vi "Get Daemon Error.vi"(8 "error in (no error)":errorcluster, 11 "Modbus slave in":refnum<class "Modbus Slave.lvclass">) -> (0 "error out":errorcluster, 2 "daemon error":errorcluster, 3 "Modbus Slave out":refnum<class "Modbus Slave.lvclass">)   [LabVIEW 2013, in "Modbus Library - Advance.lvlib" / "Modbus Slave.lvclass"]
doc: "This VI is an accessor for the <B>daemon error</B> stored in the Modbus slave instance. This accessor can be used as a property node. This status indicates the error state of the Modbus daemon."
uses:
  Modbus Slave.lvclass
  Modbus Slave.lvclass/Modbus Slave.ctl
  Network Protocol/Network Slave/Network Slave.lvclass
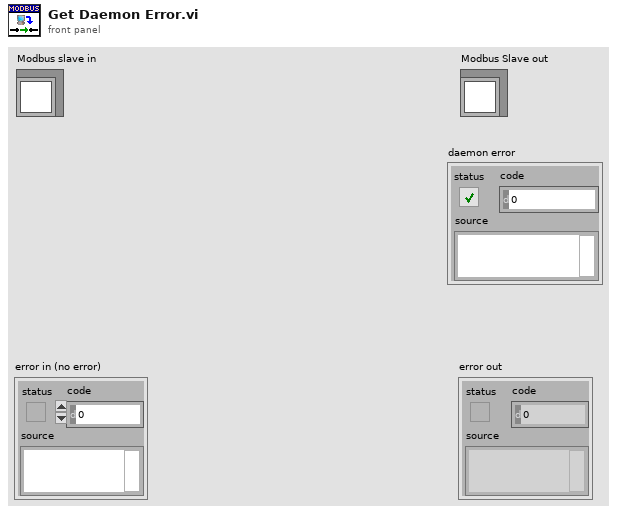
[diagram p1: front panel]
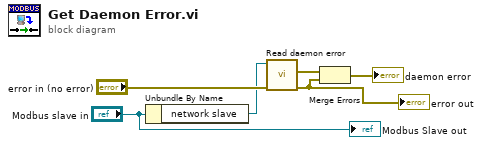
[diagram p0: block diagram]
diagram:
  n1 = Unbundle By Name("Modbus slave in") -> ("network slave"=w1:refnum<class "Network Slave.lvclass">)
  n2 = call "Read daemon error.vi"("error in (no error)"="error in (no error)", "Network Slave in"=w1) -> ("error out"=w4:errorcluster, "daemon error"=w3:errorcluster)  [unwired: 7 in, 1 out]
  "error out" <- w4
  n3 = Merge Errors(w3, w4) -> (→"daemon error":errorcluster)
  "Modbus Slave out" <- "Modbus slave in"
